vi "test - List SysLevel CSM Modules.vi"(8 "error in (no error)":errorcluster, 11 "TestCase in":refnum<class "testcase-Basic-Function.lvclass">) -> (0 "error out":errorcluster, 3 "TestCase out":refnum<class "testcase-Basic-Function.lvclass">)   [LabVIEW 2017, in "testcase-Basic-Function.lvclass"]
uses:
  testcase-Basic-Function.lvclass
  testcase-Basic-Function.lvclass/testcase-Basic-Function.ctl
  src/user.lib/_NEVSTOP/Communicable State Machine(CSM)/_Support/Error/CSM Invalid Name Error.vi
  <vilib>/addons/_JKI Toolkits/VI Tester/TestCase.llb/TestCase.lvclass
  src/user.lib/_NEVSTOP/Communicable State Machine(CSM)/Communicable State Machine.lvlib
  C:/Program Files (x86)/National Instruments/LabVIEW 2017/vi.lib/addons/_JKI Toolkits/VI Tester/TestCase.llb/TestCase.lvclass
panel:
  out "error out 2":errorcluster
  out "CSM Name(marked as Sysetem-Level Module)":string
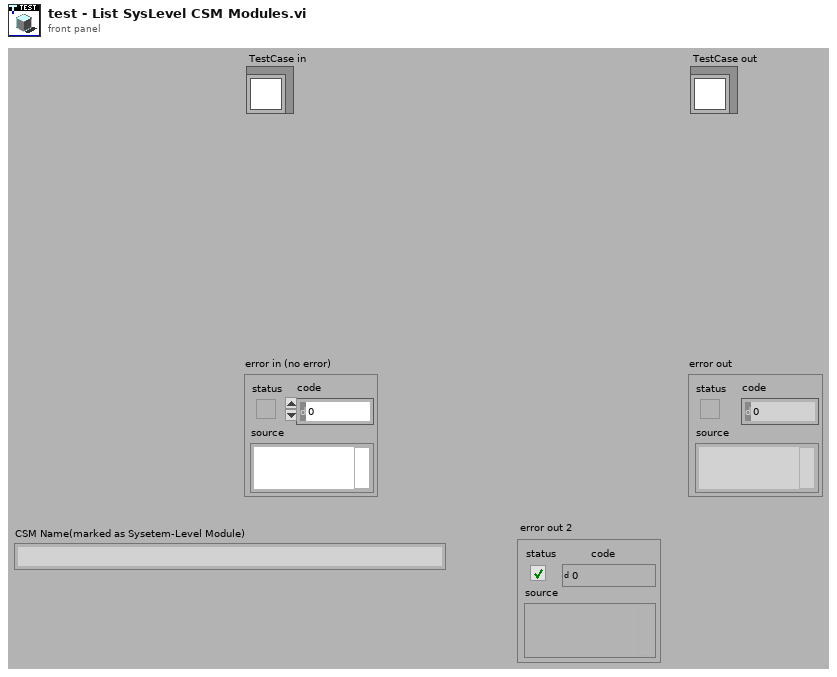
[diagram p1: front panel]
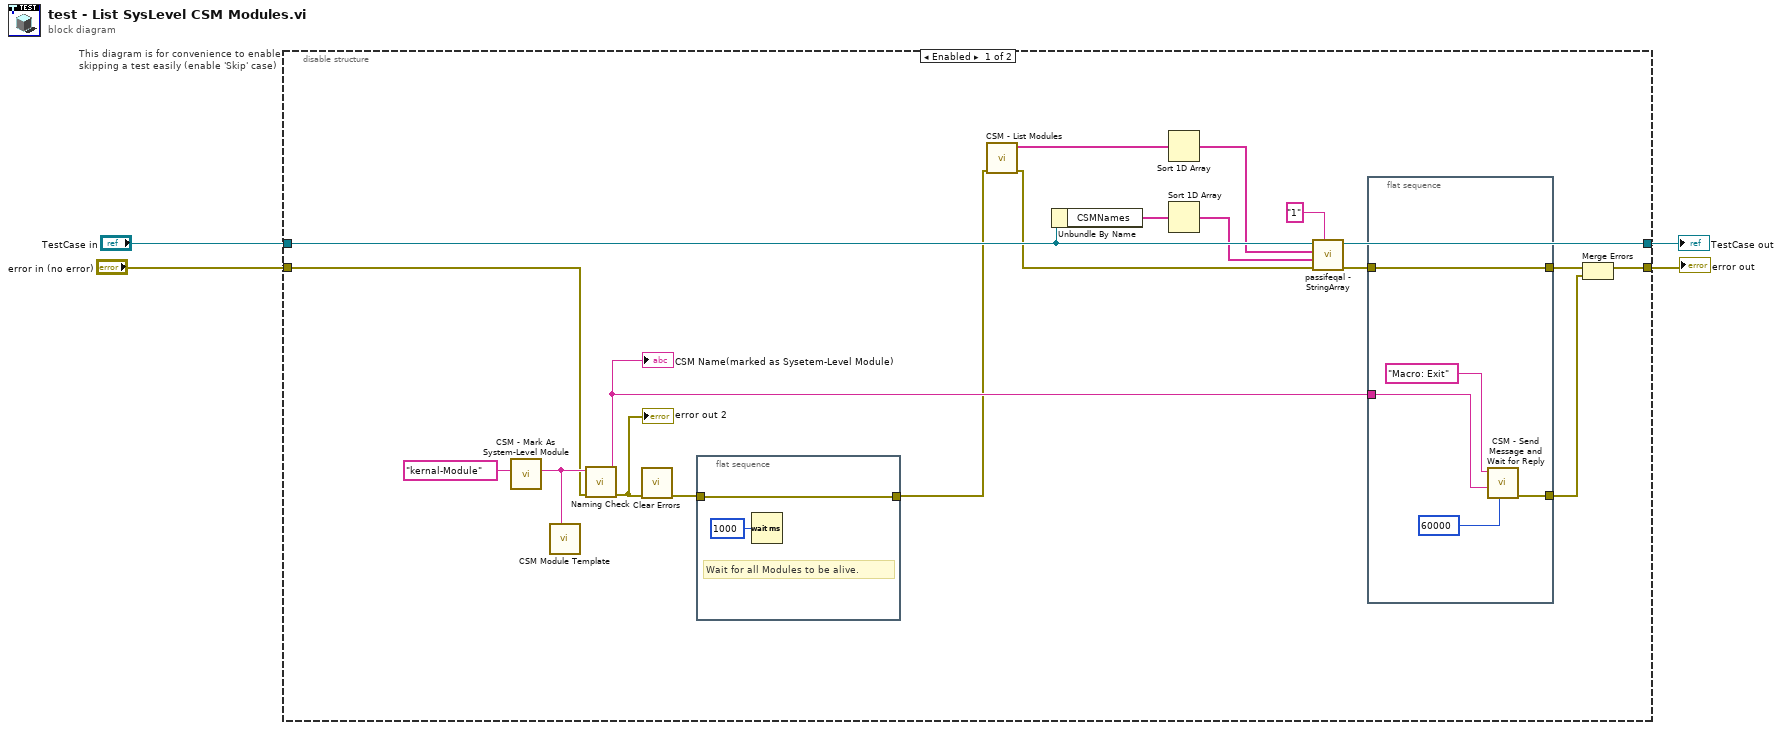
[diagram p0: block diagram]
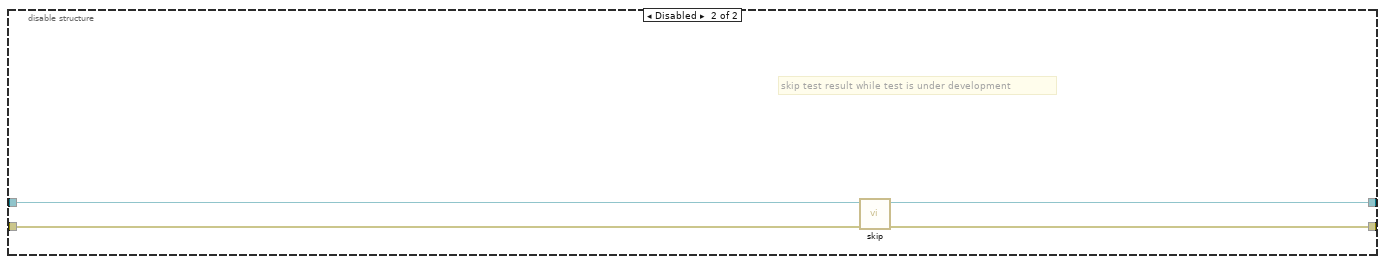
[diagram p2: hidden frame]
diagram:
  n1 = disable-structure "This diagram is for convenience to enable skipping a test easily (enable 'Skip' case)" shown="Enabled" {
    disable-tunnel: "TestCase in" -> [w21 w34]
    disable-tunnel: [w23 w32] -> w1
    disable-tunnel: [w11 w33] -> w3
    disable-tunnel: "error in (no error)" -> [w13 w31]
    frame Enabled {
      n2 = call "CSM - Mark As System-Level Module.vi"("CSM Name"="kernal-Module") -> ("CSM Name (Marked As Sysetem-Level Module)"=w17:string)  [unwired: 9 in]
      n3 = call "CSM Module Template.vi"("Name (\"\" to Use UUID)"=w17) -> ()  [unwired: 11 in]
      n4 = call "Naming Check.vi"("error in (no error)"=w13, "Name (\"\" to Use UUID)"=w17) -> ("error out"=w16:errorcluster, "Name (Dup)"=w14:string)  [unwired: 8 in]
      "CSM Name(marked as Sysetem-Level Module)" <- w14
      "error out 2" <- w16
      n5 = call <vilib>:"Clear Errors.vi"("error in (no error)"=w16) -> ("error out"=w15:errorcluster)  [unwired: 5 in, 1 out]
      n6 = flat-sequence {
        tunnel: [w29] -> w12
        tunnel: w15 -> [w29]
        frame #0 {
          # "Wait for all Modules to be alive."
          n7 = Wait (ms)(milliseconds to wait=u32 1000) -> ()  [unwired: 1 out]
        }
      }
      n8 = call "CSM - List Modules.vi"("Error In"=w12) -> ("error out"=w20:errorcluster, "Module Names"=w22:string[])  [unwired: 9 in]
      n9 = Unbundle By Name(w21) -> ("CSMNames"=w19:string[])
      n10 = Sort 1D Array(array=w22) -> (sorted array=w6:string[])
      n11 = Sort 1D Array(array=w19) -> (sorted array=w7:string[])
      n12 = call "passifeqal - StringArray.vi"("custom report message (\"\")"="1" ("custom report message (\"\")"), "error in (no error)"=w20, "y"=w7, "x"=w6, "testcase-Basic-Function in"=w21) -> ("error out"=w8:errorcluster, "testcase-Basic-Function out"=w23:refnum<class "testcase-Basic-Function.lvclass">)  [unwired: 4 in]
      n13 = flat-sequence {
        tunnel: w14 -> [w28]
        tunnel: [w26] -> w10
        tunnel: [w25] -> w9
        tunnel: w8 -> [w25]
        frame #0 {
          n14 = call "CSM - Send Message and Wait for Reply.vi"("Response Timeout (-2 Using Global Settings)"=60000, "Target Module"=w28, "State"="Macro: Exit" ("CSM Name")) -> ("error out"=w26:errorcluster)  [unwired: 6 in, 2 out]
        }
      }
      n15 = Merge Errors(w9, w10) -> (w11:errorcluster)
    }
    frame Disabled {
      # "skip test result while test is under development"
      n16 = call <vilib>:"skip.vi"("error in (no error)"=w31, "TestCase in"=w34) -> ("error out"=w33:errorcluster, "TestCase out"=w32:refnum<class "testcase-Basic-Function.lvclass">)  [unwired: 8 in]
    }
  }
  "error out" <- w3
  "TestCase out" <- w1
